vi "ArduinoOpen.vi"(8 "error in (no error)":errorcluster, 11 "ArduinoControl in":refnum<class "ArduinoControl.lvclass">) -> (0 "error out":errorcluster, 3 "ArduinoControl out":refnum<class "ArduinoControl.lvclass">)   [LabVIEW 2013, in "ArduinoControl.lvclass"]
uses:
  ArduinoControl.lvclass
  ArduinoControl.lvclass/ArduinoControl.ctl
  InstrumentSetup.vi
  <vilib>/Instr/_visa.llb/VISA Configure Serial Port (Instr).vi
  InstrControl.lvclass
panel:
  in  "Enable Termination\nChar (T)":bool=TRUE
  in  "termination char\n(0xA = '\\n' = LF)":u8=10 format="%.0x"
  in  "baud rate (9600)":u32=9600
  in  "Max number timeouts":u32=20
  out "VISA resource name out":refnum<visa-resource-name>
  out "Moin, moin!":string
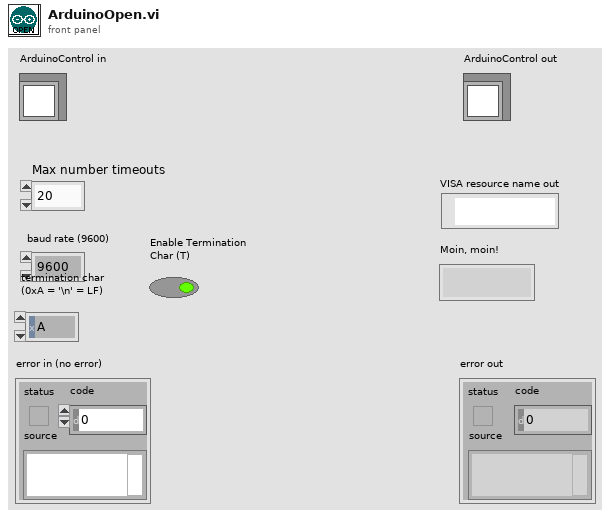
[diagram p1: front panel]
types:
  T1 = cluster{"VISA address":refnum<visa-resource-name>, "T sensor":enum16{"SHT", "DS"}, "Arduino":refnum<class "ArduinoControl.lvclass">}
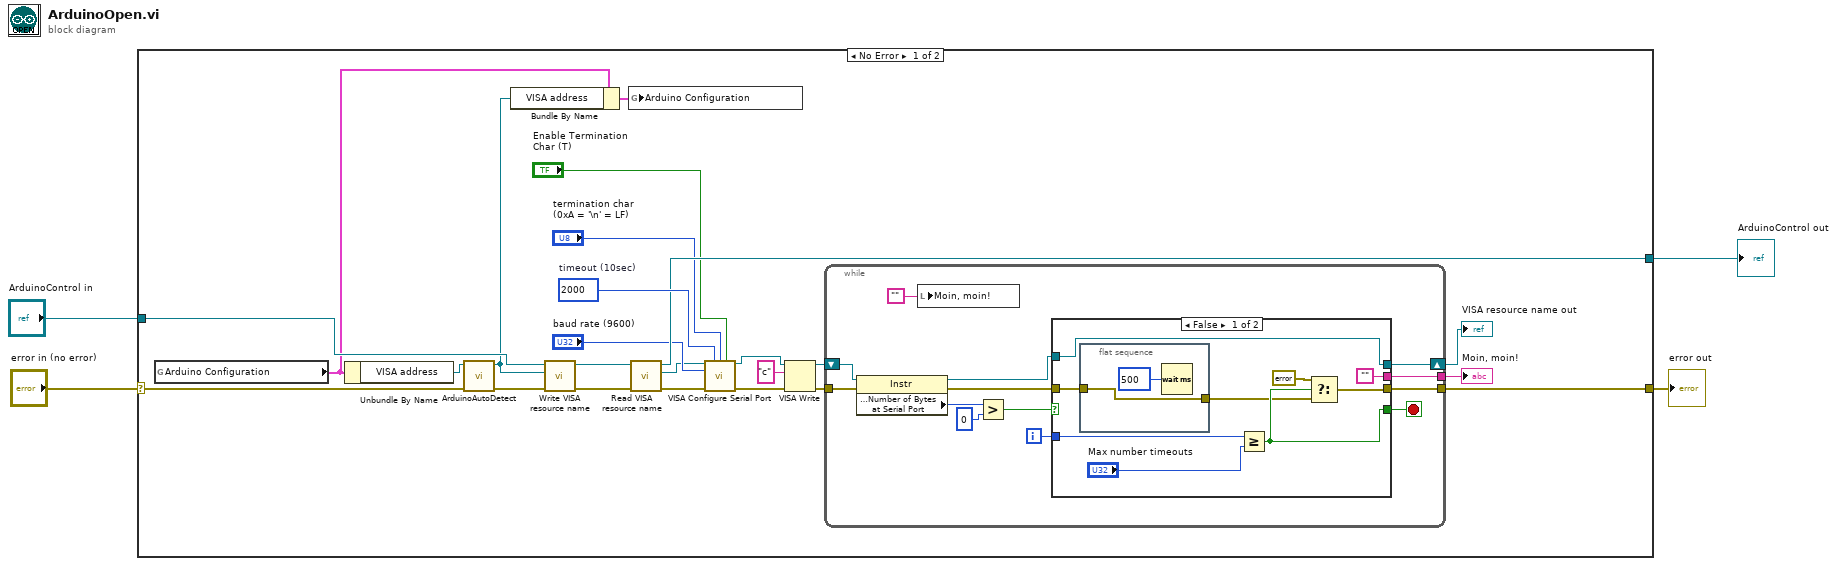
[diagram p0: block diagram]
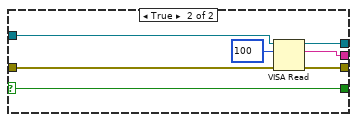
[diagram p2: hidden frame]
diagram:
  n1 = case shown="No Error" "error in (no error)" {
    selector: "error in (no error)" -> [w14 w61]
    tunnel: [w25 w61] -> w3
    tunnel: [w16 w60] -> w1
    tunnel: "ArduinoControl in" -> [w23 w60]
    frame No Error {
      w20 = u32 2000  # timeout (10sec)
      n2 = global read "InstrumentSetup.vi" "Arduino Configuration"() -> (w11:T1)
      n3 = Unbundle By Name(w11) -> ("VISA address"=w15:refnum<visa-resource-name>)
      n4 = call "ArduinoAutoDetect.vi"("error in (no error)"=w14, "Visa Resource"=w15) -> ("error out"=w13:errorcluster, "VISA resource"=w10:refnum<visa-resource-name>)  [unwired: 8 in]
      n5 = Bundle By Name(cluster=w11, "VISA address"=w10) -> (w12:T1)
      n6 = call "Write VISA resource name.vi"("error in (no error)"=w13, "VISA resource name"=w10, "ArduinoControl in"=w23) -> ("error out"=w21:errorcluster, "ArduinoControl out"=w22:refnum<class "ArduinoControl.lvclass">)  [unwired: 7 in]
      n7 = global write "InstrumentSetup.vi" "Arduino Configuration"(w12) -> ()
      n8 = call "Read VISA resource name.vi"("error in (no error)"=w21, "ArduinoControl in"=w22) -> ("error out"=w6:errorcluster, "VISA resource name"=w5:refnum<visa-resource-name>, "ArduinoControl out"=w16:refnum<class "ArduinoControl.lvclass">)  [unwired: 7 in]
      n9 = call-poly "VISA Configure Serial Port"("VISA resource name"=w5, "timeout (10sec)"=w20, "termination char\n(0xA = '\\n' = LF)"="termination char\n(0xA = '\\n' = LF)", "Enable Termination\nChar (T)"="Enable Termination\nChar (T)", "baud rate (9600)"="baud rate (9600)", "error in (no error)"=w6) -> ("VISA resource name out"=w19:refnum<visa-resource-name>, "error out"=w18:errorcluster)  [unwired: 8 in]
      n10 = VISA Write(VISA resource name=w19, write buffer="c", error in (no error)=w18) -> (VISA resource name out=w26:refnum<visa-resource-name>, error out=w28:errorcluster)  [unwired: 1 out]
      n11 = while {
        shift-right: [w36] -> w24
        shift-left: w26 -> [w39]
        tunnel: [w35] -> w25
        tunnel: [w34] -> w27
        tunnel: w28 -> [w33]
        i -> [w29]
        stop <- w30 stop-if-true
        n12 = property class="Instr"(reference=w39, error in=w33) -> (reference out=w38:refnum<visa-resource-name>, error out=w32:errorcluster, "Serial Settings:Number of Bytes at Serial Port"=w41:u32)
        n13 = local write "Moin, moin!"("") -> ()
        n14 = Greater?(x=w41, y=0) -> (0:w37:bool)
        n15 = case shown="False" w37 {
          selector: w37 -> [_ w53]
          tunnel: w38 -> [w43 w59]
          tunnel: [w43 w58] -> w36
          tunnel: [w46 w57] -> w35
          tunnel: ["" w56] -> w34
          tunnel: w32 -> [w42 w55]
          tunnel: [w45 w53] -> w30
          tunnel: w29 -> [w48 _]
          frame False {
            n16 = flat-sequence {
              tunnel: [w51] -> w44
              tunnel: w42 -> [w51]
              frame #0 {
                n17 = Wait (ms)(milliseconds to wait=u32 500) -> ()  [unwired: 1 out]
              }
            }
            n18 = Greater Or Equal?(x=w48, y="Max number timeouts") -> (x >= y?=w45:bool)
            n19 = Select(t=errorcluster {"status"=TRUE, "code"=5002, "source"="Init.vi.  Unable to establish connection with Arduino.  Please ensure that you have selected the correct COM port and that you have flashed the Arduino with the correct firmware."} ("error out"), s=w45, f=w44) -> (s? t:f=w46:errorcluster)
          }
          frame True {
            n20 = VISA Read(VISA resource name=w59, byte count=100, error in (no error)=w55) -> (VISA resource name out=w58:refnum<visa-resource-name>, read buffer=w56:string, error out=w57:errorcluster)  [unwired: 1 out]
          }
        }
      }
      "Moin, moin!" <- w27
      "VISA resource name out" <- w24
    }
    frame Error {
    }
  }
  "error out" <- w3
  "ArduinoControl out" <- w1
